vi "Read Session Present.vi"(8 "error in (no error)":errorcluster, 11 "CONNACK in":refnum<class "CONNACK.lvclass">) -> (0 "error out":errorcluster, 2 "Session Present":bool, 3 "CONNACK out":refnum<class "CONNACK.lvclass">)   [LabVIEW 2013, in "CONNACK.lvclass"]
uses:
  CONNACK.lvclass
  ControlPacket/ControlPacket.lvclass/ControlPacket.ctl
  ControlPacket/ControlPacket.lvclass
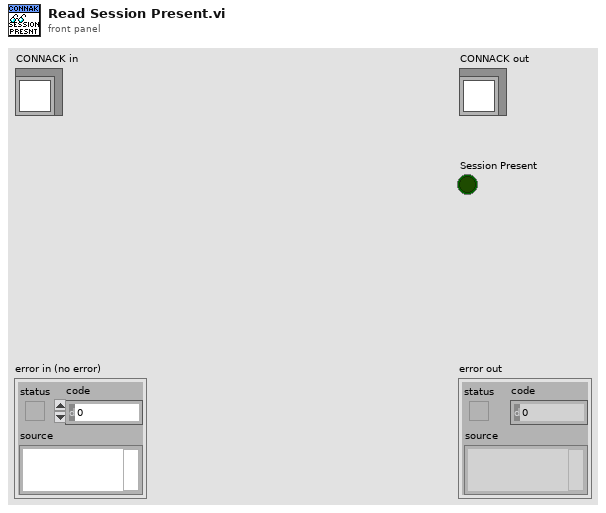
[diagram p1: front panel]
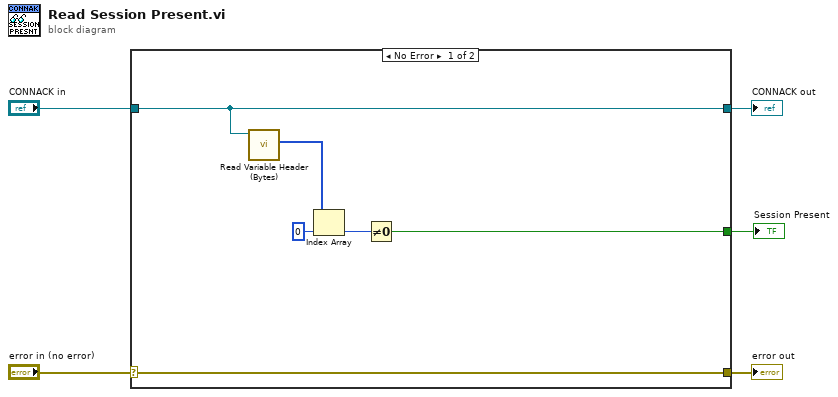
[diagram p0: block diagram]
diagram:
  n1 = case shown="No Error" "error in (no error)" {
    selector: "error in (no error)" -> [w11 w13]
    tunnel: [w11 w13] -> w4
    tunnel: [w10 w12] -> w2
    tunnel: "CONNACK in" -> [w10 w12]
    tunnel: [w6 _] -> w1
    frame No Error {
      n2 = call "Read Variable Header (Bytes).vi"("ControlPacket in"=w10) -> ("Variable Header (Bytes)"=w9:u8[])  [unwired: 9 in, 1 out]
      n3 = Index Array(array=w9, index=0) -> (element=w7:u8)
      n4 = Not Equal To 0?(x=w7) -> (x != 0?=w6:bool)
    }
    frame Error {
    }
  }
  "error out" <- w4
  "CONNACK out" <- w2
  "Session Present" <- w1
